vi "Camera_host.vi"() -> ()   [LabVIEW 2017]
uses:
  <vilib>/vision/Image Controls.llb/IMAQ Image.ctl
  <vilib>/userdefined/High Color/IMAQdx.ctl
  <vilib>/vision/Avi.llb/IMAQ AVI2 Refnum.ctl
  camera_array_1.ctl
  <vilib>/vision/Avi.llb/IMAQ AVI2 Codec Path.ctl
  Globals/Global - Configuration Options.vi
  <vilib>/vision/driver/NI_Vision_Acquisition_Software.lvlib
panel:
  in  "Boolean":bool
  out "Array":T1[](array[typedef])
  out "Webcam":T1(plugin-control)
  out "Codec Names 2":string[](array[string])
  out "concatenated string 4":string
  out "error out":errorcluster
  out "x-y":u32
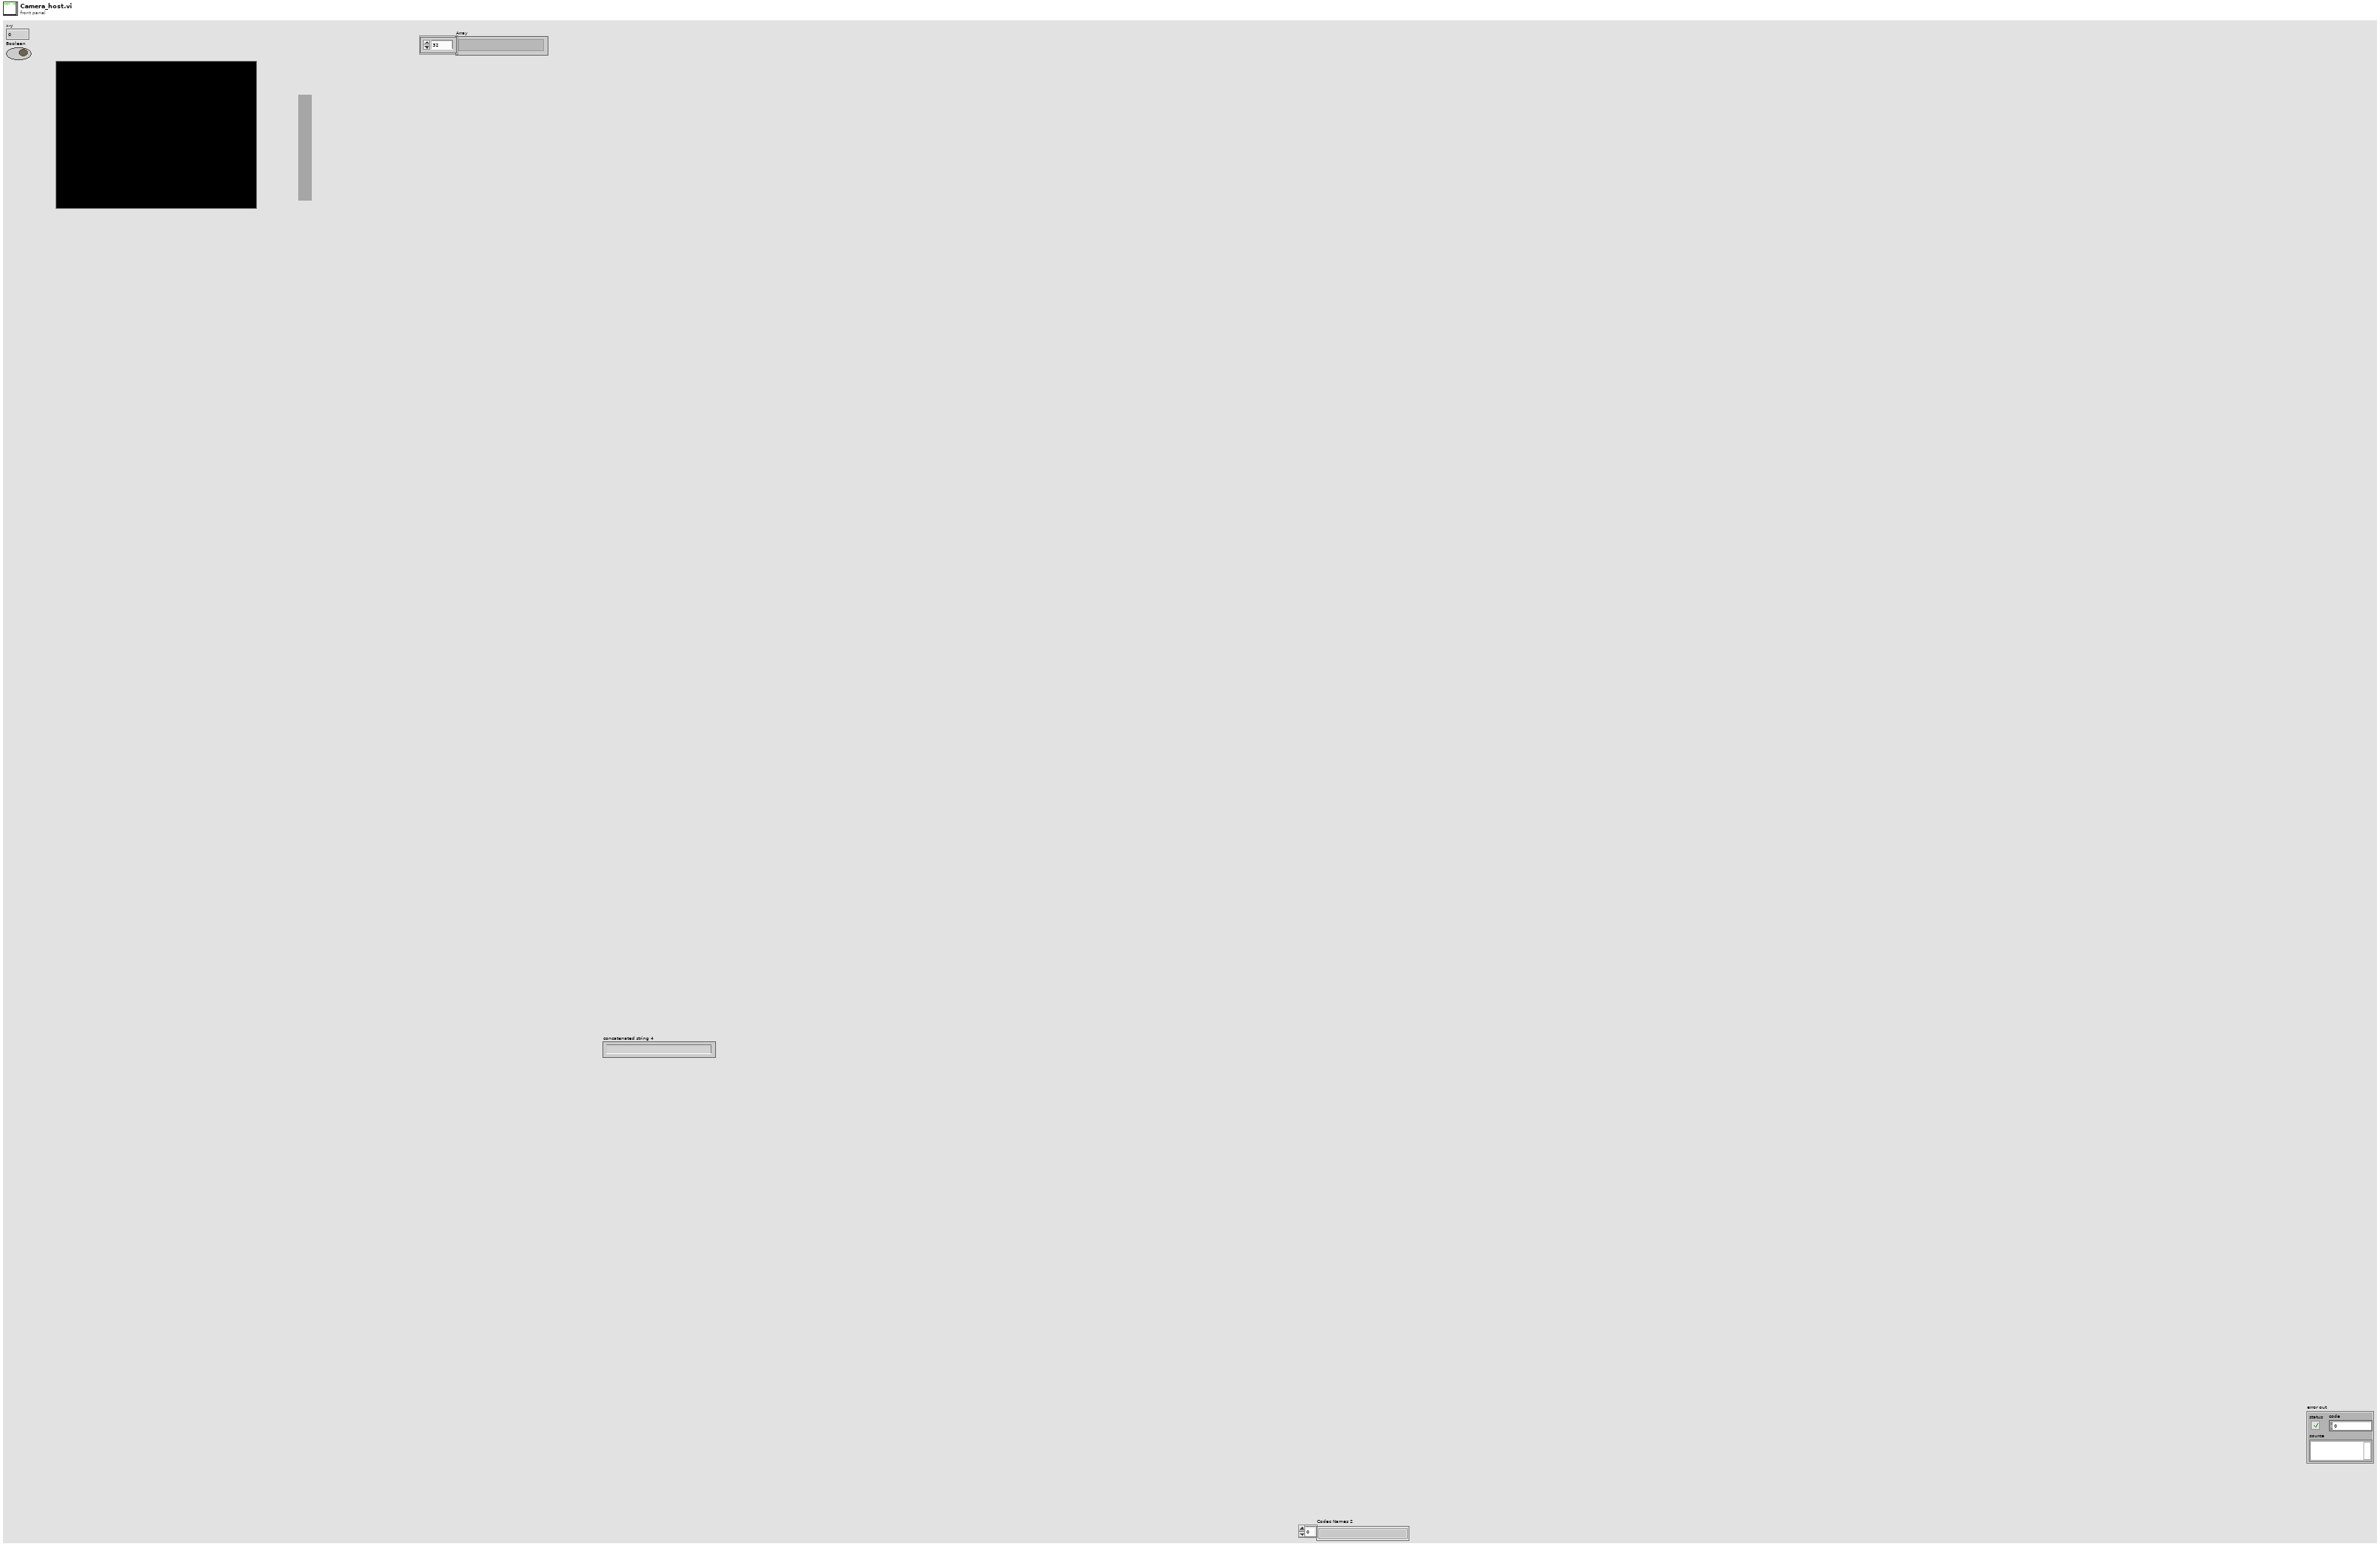
[diagram p1: front panel]
types:
  T1 = typedef "IMAQ Image.ctl" = refnum<image>
  T2 = typedef "camera_array_1.ctl" = T1[]
  T3 = typedef "IMAQ AVI2 Refnum.ctl" = refnum<k20>
  T4 = typedef "IMAQdx.ctl" = refnum<k21>
  T5 = typedef "Image Type" = u32
  T6 = cluster{"Tool data":cluster{"Number of teeth":sgl}, "Cutting data":cluster{"rpm":sgl}, "Limits":cluster{"Magnitude threshold":sgl, "Tolerance":sgl}, "G1 status":cluster{"G1 trigger":bool}}
  T7 = typedef "IMAQ AVI2 Codec Path.ctl" = u32
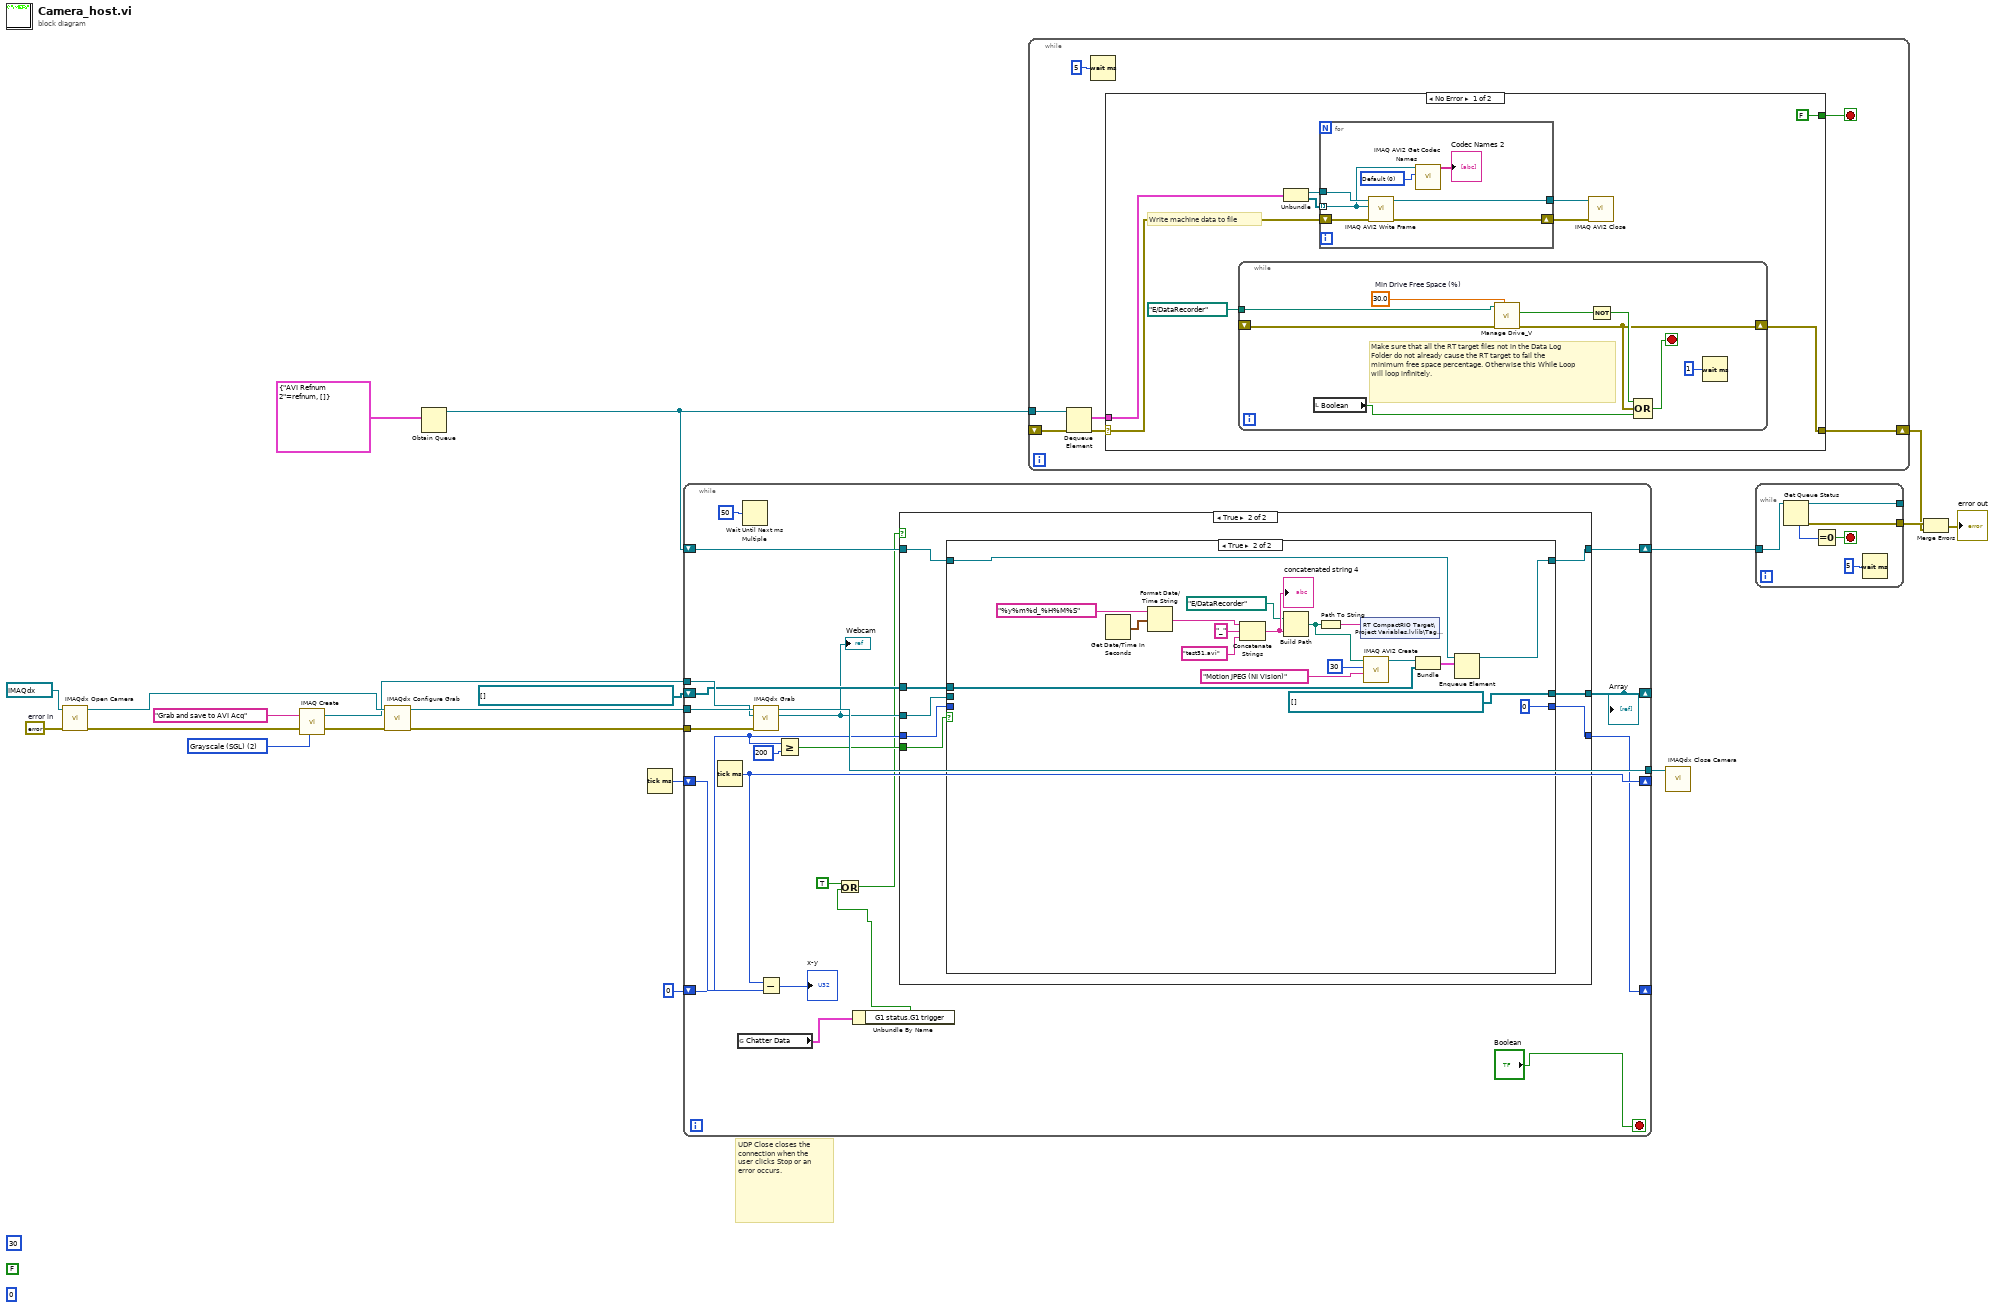
[diagram p0: block diagram]
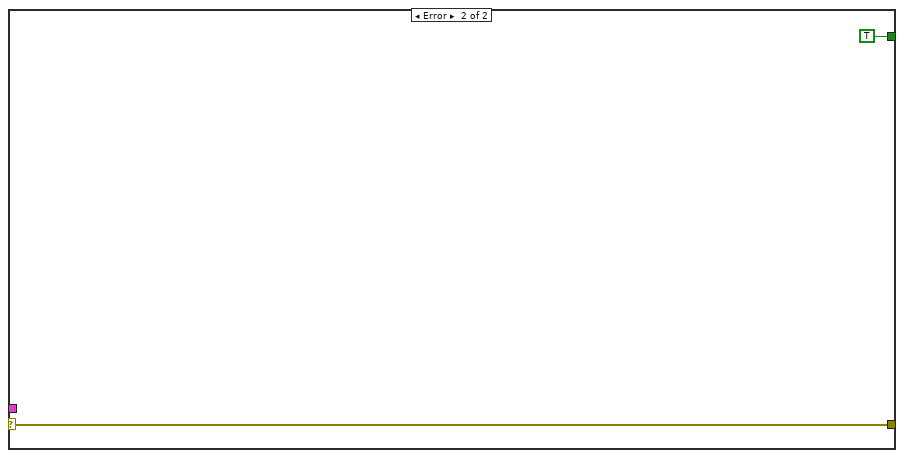
[diagram p2: hidden frame]
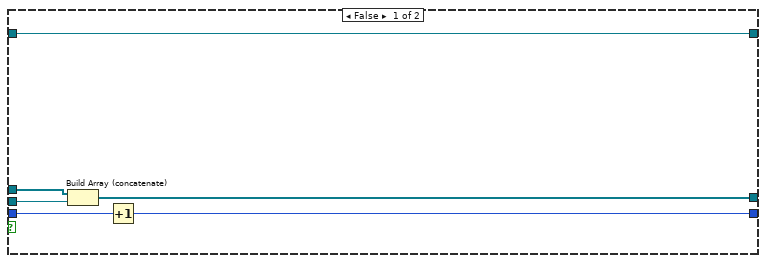
[diagram p4: hidden frame]
diagram:
  w11 = T5 2 items=["Grayscale (U8)", "Grayscale (I16)", "Grayscale (SGL)", "Complex (CSG)", "RGB (U32)", "HSL (U32)", "RGB (U64)", "Grayscale (U16)"] ("Image Type")
  (unwired) u32 30 ("Frames Per Second")
  w12 = errorcluster {"status"=FALSE, "code"=0, "source"=""}  # error in
  (unwired) i16 0 ("A(I16) 11")
  (unwired) FALSE
  # "UDP Close closes the connection when the user clicks Stop or an error occurs."
  n1 = call <vilib>:"IMAQdx Open Camera.vi"("error in"=w12, "Session In"=T4 "cam0") -> ("error out"=w10:errorcluster, "Session Out"=w14:T4)  [unwired: 8 in]
  n2 = call "IMAQ Create"("Image Name"="Grab and save to AVI Acq", "Image Type"=w11, "error in (no error)"=w10) -> ("New Image"=w7:T1, "error out"=w6:errorcluster)  [unwired: 2 in]
  n3 = call <vilib>:"IMAQdx Configure Grab.vi"("error in"=w6, "Session In"=w14) -> ("error out"=w5:errorcluster, "Session Out"=w8:T4)  [unwired: 8 in]
  n4 = Obtain Queue(element data type=cluster{"AVI Refnum 2":T3, T1[]} {"AVI Refnum 2"=refnum, []}) -> (queue out=w18:refnum<queue>)  [unwired: 4 in, 2 out]
  n5 = Tick Count (ms)() -> (millisecond timer value=w15:u32)
  n6 = while {
    shift-right: [w41] -> w20
    shift-left: w18 -> [w42]
    shift-right: [w38] -> _
    shift-left: w15 -> [w39]
    tunnel: w8 -> [w37]
    tunnel: w7 -> [w36]
    tunnel: w5 -> [w35]
    tunnel: [w34] -> w4
    shift-right: [w27] -> _
    shift-left: T2 [] -> [w31]
    shift-right: [w28] -> _
    shift-left: 0 -> [w29]
    stop <- "Boolean" stop-if-true
    n7 = Tick Count (ms)() -> (millisecond timer value=w38:u32)
    n8 = global read "Global - Configuration Options.vi" "Chatter Data"() -> (w21:T6)
    n9 = Wait Until Next ms Multiple(millisecond multiple=u32 50) -> ()  [unwired: 1 out]
    n10 = call <vilib>:"IMAQdx Grab.vi"("error in"=w35, "Image In"=w36, "Session In"=w37) -> ("Image Out"=w26:T1, "Session Out"=w34:T4)  [unwired: 5 in, 2 out]
    "Webcam" <- w26
    n11 = Subtract(x=w38, y=w39) -> (x-y=→"x-y":u32)
    n12 = Greater Or Equal?(x=w29, y=200) -> (x >= y?=w30:bool)
    n13 = Unbundle By Name(w21) -> ("G1 status.G1 trigger"=w25:bool)
    n14 = Or(x=TRUE, y=w25) -> (x .or. y?=w23:bool)
    n15 = case shown="True" w23 {
      tunnel: w42 -> [w45 w46]
      tunnel: [w45 w53] -> w41
      tunnel: w26 -> [_ w52]
      tunnel: w31 -> [w43 w50]
      tunnel: w30 -> [_ w51]
      tunnel: w29 -> [w44 w49]
      tunnel: [w44 w48] -> w28
      tunnel: [w43 w47] -> w27
      frame False {
      }
      frame True {
        n16 = case shown="True" w51 {
          tunnel: [w56 w64] -> w53
          tunnel: w52 -> [w58 _]
          tunnel: w50 -> [w59 w62]
          tunnel: w49 -> [w57 _]
          tunnel: [w55 0] -> w48
          tunnel: [w54 T1[] []] -> w47
          tunnel: w46 -> [w56 w65]
          frame False {
            n17 = Build Array (concatenate)(w59, w58) -> (w54:T2)
            n18 = Increment(x=w57) -> (x+1=w55:i32)
          }
          frame True {
            n19 = Get Date/Time In Seconds() -> (seconds since 1Jan1904=w74:timestamp)
            n20 = Format Date/Time String(time format string (%c)="%y%m%d_%H%M%S", seconds (now)=w74) -> (date/time string=w75:string)  [unwired: 1 out]
            n21 = Concatenate Strings(w75, "_" ("string"), "test51.avi" ("name or relative path")) -> (w76:string)
            "concatenated string 4" <- w76
            n22 = Build Path(base path=path "E:/DataRecorder" ("AVI Path"), name or relative path=w76) -> (appended path=w67:path)
            n23 = Path To String(path=w67) -> (string=w77:string)
            n24 = shared-variable "RT CompactRIO Target\\Project Variables.lvlib\\Tag Video"(w77) -> ()  [unwired: 1 in, 1 out]
            n25 = call "IMAQ AVI2 Create"("Codec"="Motion JPEG (NI Vision)", "Frames Per Second"=u32 30, "AVI Path"=w67) -> ("AVI Refnum"=w63:T3)  [unwired: 7 in, 1 out]
            n26 = Bundle("AVI Refnum"=w63, w62) -> (w61:cluster{"AVI Refnum":T3, T2})  [unwired: 1 in]
            n27 = Enqueue Element(queue=w65, element=w61) -> (queue out=w64:refnum<queue>)  [unwired: 2 in, 2 out]
          }
        }
      }
    }
    "Array" <- w27
  }
  n28 = while {
    tunnel: w18 -> [w84]
    shift-right: [w80] -> w17
    shift-left: _ -> [w83]
    stop <- w81 stop-if-true
    n29 = Dequeue Element(queue=w84, error in (no error)=w83) -> (element=w79:cluster{"AVI Refnum 2":T3, T1[]}, error out=w82:errorcluster)  [unwired: 1 in, 2 out]
    n30 = Wait (ms)(milliseconds to wait=u32 5) -> ()  [unwired: 1 out]
    n31 = case shown="No Error" w82 {
      selector: w82 -> [w92 w110]
      tunnel: [FALSE TRUE] -> w81
      tunnel: [w88 w110] -> w80
      tunnel: w79 -> [w87 _]
      frame No Error {
        # "Write machine data to file"
        n32 = while {
          shift-right: [w105] -> w88
          shift-left: _ -> [w106]
          tunnel: path "E:/DataRecorder" ("AVI Path") -> [w103]
          stop <- w109 stop-if-true
          w104 = 30.0  # Min Drive Free Space (%)
          # "Make sure that all the RT target files not in the Data Log Folder do not already cause the RT target to fail the minimum free space percentage. Otherwise this While Loop will loop infinitely."
          n33 = local read "Boolean"() -> (w101:bool)
          n34 = call "Manage Drive_V.vi"("Min Drive Free Space (%)"=w104, "error in"=w106, "Data Folder"=w103) -> ("error out"=w105:errorcluster, "Drive Space Below Limit"=w102:bool)  [unwired: 6 in, 1 out]
          n35 = Not(x=w102) -> (.not. x?=w108:bool)
          n36 = Compound Arithmetic op=OR(w108, w105, w101) -> (w109:bool)
          n37 = Wait (ms)(milliseconds to wait=u32 1) -> ()  [unwired: 1 out]
        }
        n38 = Unbundle(w87) -> ("AVI Refnum 2"=w86:T3, w85:T1[])
        n39 = for {
          shift-right: [w98] -> w90
          shift-left: w92 -> [w100]
          tunnel: w86 -> [w97]
          tunnel: [w99] -> w91
          tunnel: w85 -> [w94] mode=indexing
          w96 = T7 0 items=["Default", "System", "Built in Vision"] ("Codec Source")
          n40 = call "IMAQ AVI2 Write Frame"("error in (no error)"=w100, "Image"=w94, "AVI Refnum"=w97) -> ("error out"=w98:errorcluster, "AVI Refnum (duplicate)"=w99:T3)  [unwired: 6 in, 1 out]
          n41 = call "IMAQ AVI2 Get Codec Names"("Codec Source"=w96, "Image"=w94) -> ("Codec Names"=→"Codec Names 2":string[])  [unwired: 8 in, 1 out]
        }
        n42 = call "IMAQ AVI2 Close"("error in (no error)"=w90, "AVI Refnum"=w91) -> ()  [unwired: 9 in, 1 out]
      }
      frame Error {
      }
    }
  }
  n43 = call <vilib>:"IMAQdx Close Camera.vi"("Session In"=w4) -> ()  [unwired: 10 in, 1 out]
  n44 = while {
    tunnel: [w116] -> w19
    tunnel: [w114] -> _
    tunnel: w20 -> [w112]
    stop <- w115 stop-if-true
    n45 = Get Queue Status(queue=w112) -> (queue out=w114:refnum<queue>, error out=w116:errorcluster, # elements in queue=w113:i32)  [unwired: 2 in, 5 out]
    n46 = Equal To 0?(x=w113) -> (x = 0?=w115:bool)
    n47 = Wait (ms)(milliseconds to wait=u32 5) -> ()  [unwired: 1 out]
  }
  n48 = Merge Errors(w19, w17) -> (→"error out":errorcluster)
